vi "Stop_Control.vi"() -> (1 "Will Stop ?":bool)   [LabVIEW 2014]
uses:
  CustomControls/Program_States.ctl
  CustomControls/TSE_Status.ctl
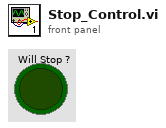
[diagram p1: front panel]
types:
  T1 = typedef "Program_States.ctl" = enum16{"Ön Yükleme", "TSE Baslat", "Kalibratöre Baglan", "Kalibratörü Baslat", "Ön Yükleme Tamam", "Frekans Testi", "Gerilim Testi", "Akim Testi", "Aktif Guc Testi", "Reaktif Guc Testi", "AC Akim Harmonik Testi", "AC Gerilim Harmonik Testi", "Flicker Testi", "Rapor Cikarma", "Yeniden Başlat", "Bekleme", "Durdur"}
  T2 = typedef "TSE_Status.ctl" = cluster{"Return Code":i32, "Message":string, "error in (no error)":errorcluster, "Program State":T1, "Test A. Suresi":u32}
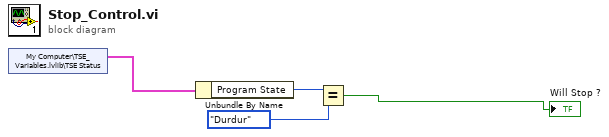
[diagram p0: block diagram]
diagram:
  n1 = shared-variable "My Computer\\TSE_Variables.lvlib\\TSE Status"() -> (w1:T2)  [unwired: 1 in, 1 out]
  n2 = Unbundle By Name(w1) -> ("Program State"=w3:T1)
  n3 = Equal?(x=w3, y=Program_States."Durdur") -> (x = y?=→"Will Stop ?":bool)
